vi "Set Setpoint.vi"(8 "error in (no error)":errorcluster, 10 "Setpoint":dbl, 11 "Lakeshore 331 in":refnum<class "Lakeshore 331.lvclass">) -> (0 "error out":errorcluster, 3 "Lakeshore 331 out":refnum<class "Lakeshore 331.lvclass">)   [LabVIEW 2022 SP3, in "Lakeshore 331.lvclass"]
uses:
  Lakeshore 331.lvclass
  Lakeshore 331.lvclass/Lakeshore 331.ctl
  Temp Control.lvclass
  <instrlib>/Lake Shore Cryotronics 331/Lake Shore Cryotronics 331.lvlib
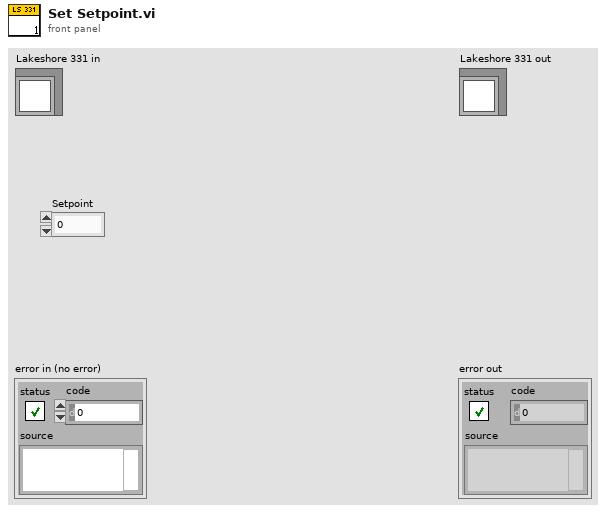
[diagram p1: front panel]
types:
  T1 = typedef "Lakeshore 331.lvclass/Lakeshore 331 Parameters.ctl" = cluster{"Mode":u16, "Setpoint":dbl, "Manual Power (%)":dbl, "Control Parameters":cluster{"P":dbl, "I":dbl, "D":u16}}
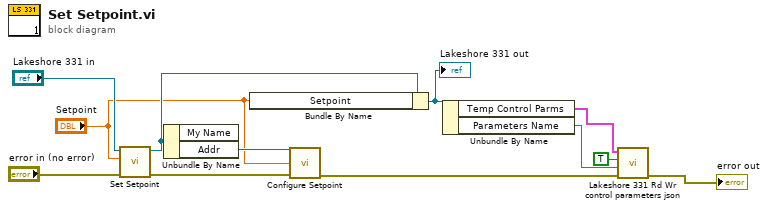
[diagram p0: block diagram]
diagram:
  n1 = call-parent "Set Setpoint.vi"("error in (no error)"="error in (no error)", "Setpoint"="Setpoint", "Temp Control in"="Lakeshore 331 in") -> ("error out"=w7:errorcluster, "Temp Control out"=w10:refnum<class "Lakeshore 331.lvclass">)  [unwired: 7 in]
  n2 = Unbundle By Name(w10) -> ("Addr"=w9:refnum<visa-resource-name>)  [unwired: 1 out]
  n3 = Bundle By Name(cluster=w10, "Setpoint"="Setpoint") -> (w4:refnum<class "Lakeshore 331.lvclass">)
  "Lakeshore 331 out" <- w4
  n4 = call <instrlib>:"Configure Setpoint.vi"("VISA resource name"=w9, "Setpoint (0.0000)"="Setpoint", "error in (no error)"=w7) -> ("error out"=w6:errorcluster)  [unwired: 11 in, 1 out]
  n5 = Unbundle By Name(w4) -> ("Temp Control Parms"=w3:T1, "Parameters Name"=w1:string)
  n6 = call "Lakeshore 331 Rd Wr control parameters json.vi"("error in (no error)"=w6, "Section"=w1, "Write? (F:Read)"=TRUE, "Temp Control Parms"=w3) -> ("error out"=→"error out":errorcluster)  [unwired: 6 in, 1 out]
